vi "Open.vi"(8 "error in (no error)":errorcluster) -> (0 "error out":errorcluster, 1 "Serial Number":string, 2 "Model":string, 3 "VISA resource name":refnum<visa-resource-name>)   [LabVIEW 2019, in "KH7008.lvlib"]
uses:
  KH7008.lvlib
  <vilib>/Instr/_visa.llb/VISA Configure Serial Port (Instr).vi
  <userlib>/LevyLab/D2XX-LV/D2XX-lv.lvlib
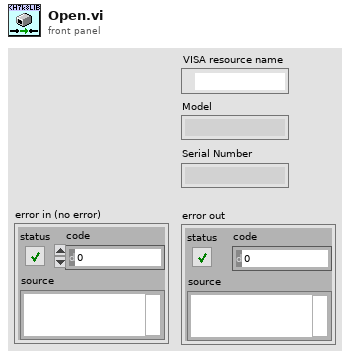
[diagram p1: front panel]
types:
  T1 = typedef "D2XX-lv.lvlib/Device Info.ctl" = cluster{"Serial Number":string, "COM port":string, "Description":string}
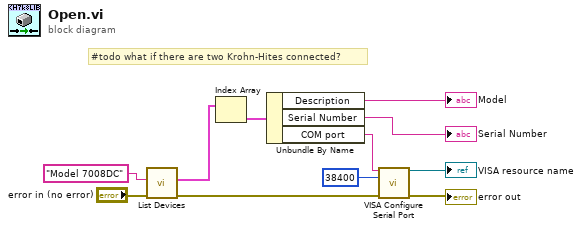
[diagram p0: block diagram]
diagram:
  # "#todo what if there are two Krohn-Hites connected?"
  n1 = call <userlib>:"List Devices.vi"("error in (no error)"="error in (no error)", "Filter (Device Description)"="Model 7008DC") -> ("error out"=w10:errorcluster, "Devices"=w8:T1[])  [unwired: 8 in]
  n2 = Index Array(array=w8) -> (element=w7:T1)  [unwired: 1 in]
  n3 = Unbundle By Name(w7) -> ("Description"=→"Model":string, "Serial Number"=→"Serial Number":string, "COM port"=w1:string)
  n4 = call-poly "VISA Configure Serial Port"("VISA resource name"=w1, "baud rate (9600)"=u32 38400, "error in (no error)"=w10) -> ("VISA resource name out"=→"VISA resource name":refnum<visa-resource-name>, "error out"=→"error out":errorcluster)  [unwired: 6 in, 5 out]
